vi "WFGenerate03PT.vi"(7 "Repetitions":T1 {"Interval (s)" min=0.0; "Delay (s)" min=0.0}, 8 "error in (no error)":errorcluster, 9 "Waveform Properties":T3 {"Ramp (s)" min=0.0; "Fs (Hz)" min=0.0}, 10 "Waveform Parameters":T2) -> (0 "error out":errorcluster, 3 "Waveform Out":waveform(dbl))   [LabVIEW 2009]
uses:
  <vilib>/measure/NI_MABase.lvlib
panel:
  out "Waveform Graph":waveform(dbl)(graph)
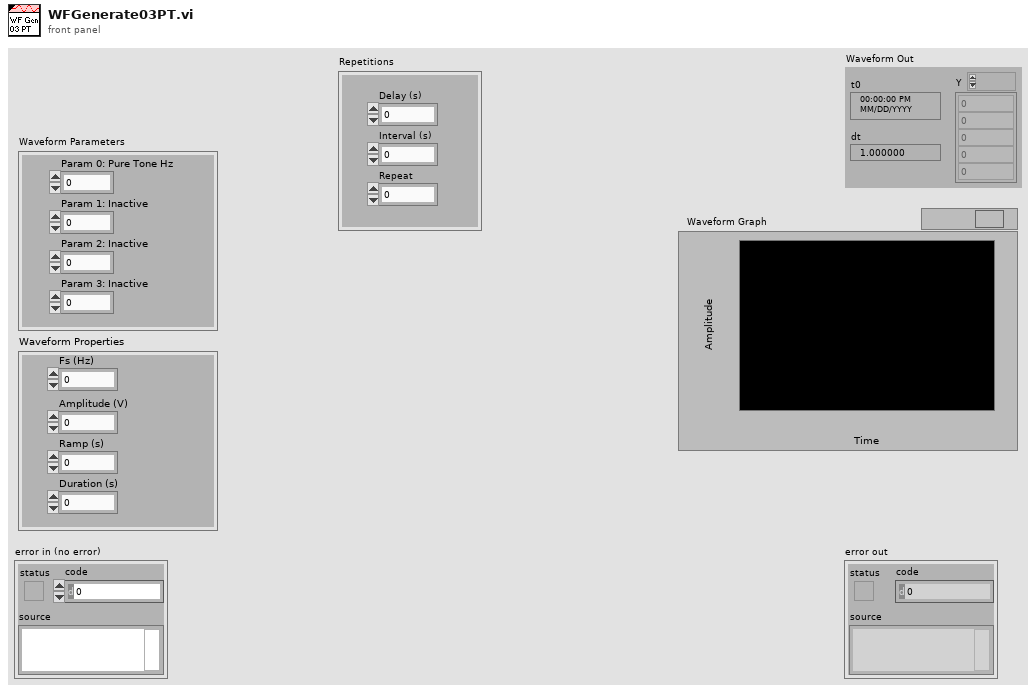
[diagram p1: front panel]
types:
  T1 = cluster{"Delay (s)":dbl, "Interval (s)":dbl, "Repeat":i32}
  T2 = cluster{"Param 0: Pure Tone Hz":dbl, "Param 1: Inactive":dbl, "Param 2: Inactive":dbl, "Param 3: Inactive":dbl}
  T3 = cluster{"Fs (Hz)":dbl, "Amplitude (V)":dbl, "Ramp (s)":dbl, "Duration (s)":dbl}
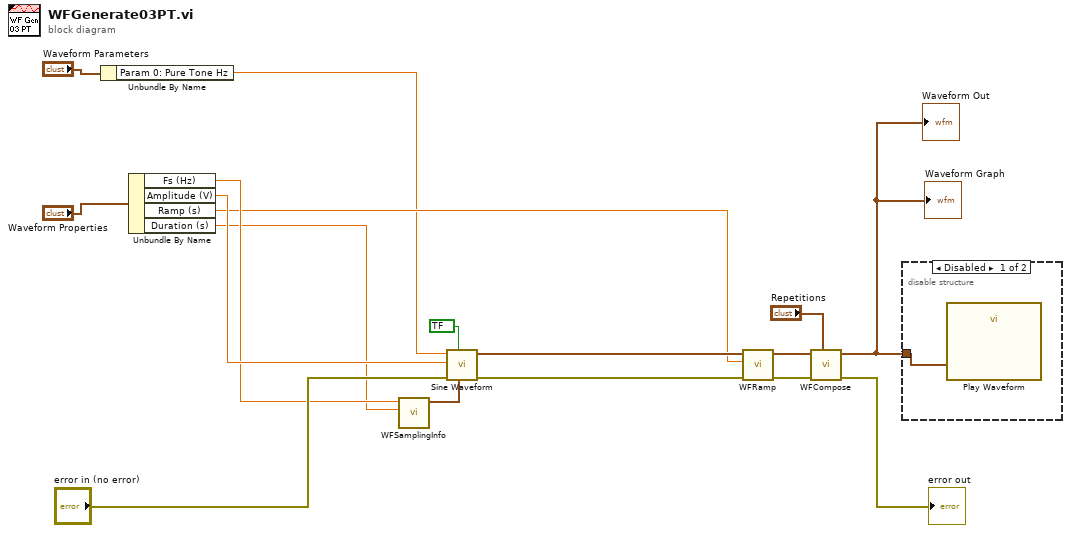
[diagram p0: block diagram]
diagram:
  n1 = Unbundle By Name("Waveform Parameters") -> ("Param 0: Pure Tone Hz"=w6:dbl)
  n2 = Unbundle By Name("Waveform Properties") -> ("Fs (Hz)"=w13:dbl, "Amplitude (V)"=w16:dbl, "Ramp (s)"=w11:dbl, "Duration (s)"=w9:dbl)
  n3 = call "WFSamplingInfo.vi"("Duration (s)"=w9, "Fs (Hz)"=w13) -> ("sampling info"=w14:cluster{"Fs":dbl, "#s":dbl})  [unwired: 9 in]
  n4 = call <vilib>:"Sine Waveform.vi"("sampling info"=w14, "reset signal"=bool ?, "error in (no error)"="error in (no error)", "amplitude"=w16, "frequency"=w6) -> ("error out"=w10:errorcluster, "signal out"=w12:waveform(dbl))  [unwired: 5 in]
  n5 = call "WFRamp.vi"("error in (no error)"=w10, "Ramp Length (s)"=w11, "Waveform In"=w12) -> ("error out"=w3:errorcluster, "Waveform Out"=w4:waveform(dbl))  [unwired: 7 in]
  n6 = call "WFCompose.vi"("Repetitions"="Repetitions", "error in (no error)"=w3, "Waveform In"=w4) -> ("error out"=→"error out":errorcluster, "Analog Waveform Out"=w1:waveform(dbl))  [unwired: 7 in]
  "Waveform Out" <- w1
  "Waveform Graph" <- w1
  n7 = disable-structure shown="Disabled" {
    disable-tunnel: w1 -> [w18 _]
    frame #0 {
      n8 = call "Play Waveform"("Data"=w18) -> ()  [unwired: 18 in, 1 out]
    }
    frame #1 {
    }
  }
